vi "Find Test Cases.vi"(8 "error in (no error)":errorcluster, 10 "Project or Class Path":path, 11 "Test Finder In":refnum<class "Test Finder.lvclass">) -> (0 "error out":errorcluster, 3 "Test Finder Out":refnum<class "Test Finder.lvclass">)   [LabVIEW 2020, in "Test Finder.lvclass"]
uses:
  Test Finder.lvclass
  Test Finder.lvclass/Test Finder.ctl
  Test Case/LUnit Test Case.lvclass
  <vilib>/Utility/error.llb/Error Cluster From Error Code.vi
  <vilib>/ErrorRing/Error Ring.xnode
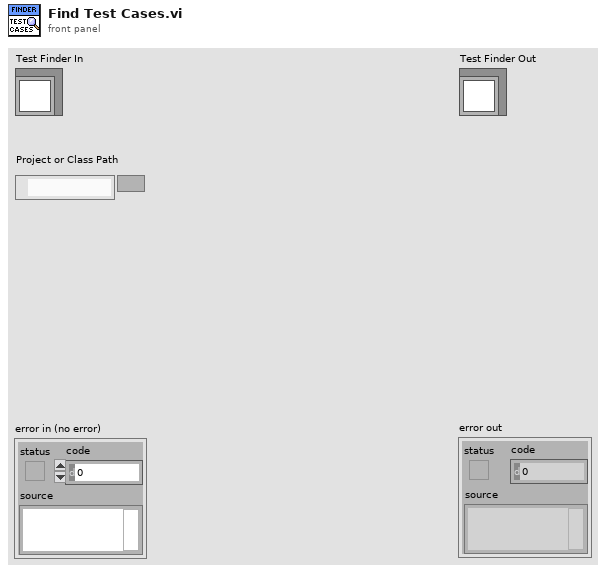
[diagram p1: front panel]
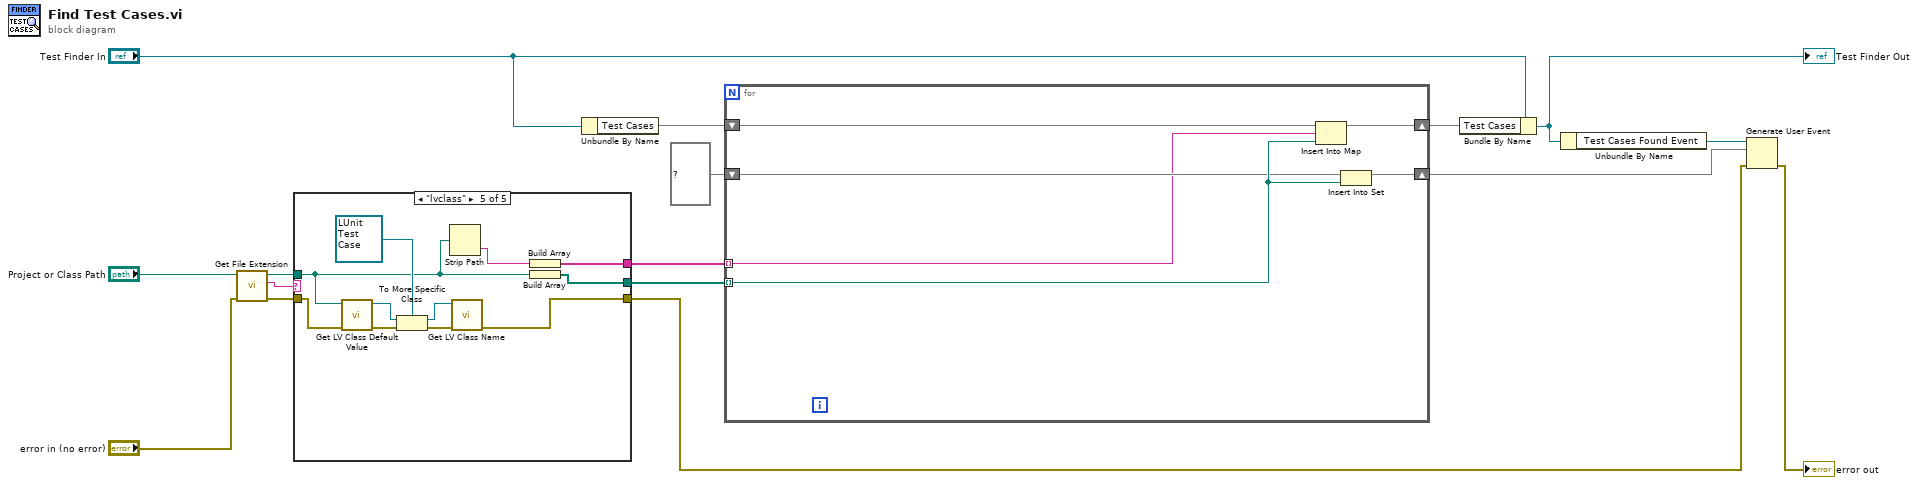
[diagram p0: block diagram]
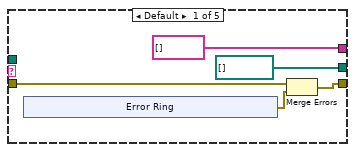
[diagram p2: hidden frame]
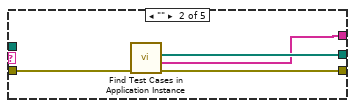
[diagram p3: hidden frame]
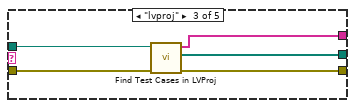
[diagram p4: hidden frame]
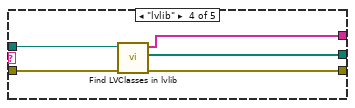
[diagram p5: hidden frame]
diagram:
  n1 = call <vilib>:"Get File Extension.vi"("error in (no error)"="error in (no error)", "file"="Project or Class Path") -> ("error out"=w13:errorcluster, "lowercase file extension"=w12:string, "dup file"=w15:path)  [unwired: 5 in, 2 out]
  n2 = case shown="\"lvclass\"" w12 {
    tunnel: w15 -> [_ _ w34 w39 w41]
    tunnel: w13 -> [w17 w27 w33 w38 w44]
    tunnel: [w18 w29 w31 w36 w43] -> w5
    tunnel: [path[] [] ("Class paths") w28 w32 w37 w50] -> w11
    tunnel: [string[] [] ("Classes in project") w26 w30 w35 w49] -> w1
    frame Default {
      n3 = xnode "Error Ring"() -> ("error out"=w21:errorcluster)
      n4 = Merge Errors(w17, w21) -> (w18:errorcluster)
    }
    frame "" {
      n5 = call "Find Test Cases in Application Instance.vi"("error in (no error)"=w27) -> ("error out"=w29:errorcluster, "Classes in App Instance"=w26:string[], "Class Paths"=w28:path[])  [unwired: 8 in]
    }
    frame "lvproj" {
      n6 = call "Find Test Cases in LVProj.vi"("error in (no error)"=w33, "Project Path"=w34) -> ("error out"=w31:errorcluster, "Class paths"=w32:path[], "Classes in project"=w30:string[])  [unwired: 7 in]
    }
    frame "lvlib" {
      n7 = call "Find LVClasses in lvlib.vi"("error in (no error)"=w38, "Library Path"=w39) -> ("error out"=w36:errorcluster, "Class paths"=w37:path[], "Classes in library"=w35:string[])  [unwired: 7 in]
    }
    frame "lvclass" {
      n8 = call <vilib>:"Get LV Class Default Value.vi"("error in (no error)"=w44, "class path"=w41) -> ("error out"=w48:errorcluster, "object"=w46:refnum<class>)  [unwired: 8 in]
      n9 = To More Specific Class(target class=refnum<class "LUnit Test Case.lvclass"> refnum ("LUnit Test Case.lvclass"), reference=w46, error in=w48) -> (specific class reference=w45:refnum<class "LUnit Test Case.lvclass">, error out=w47:errorcluster)
      n10 = Strip Path(path=w41) -> (name=w40:string)  [unwired: 1 out]
      n11 = call <vilib>:"Get LV Class Name.vi"("error in (no error)"=w47, "object"=w45) -> ("error out"=w43:errorcluster)  [unwired: 8 in, 1 out]
      n12 = Build Array(w40) -> (w49:string[])
      n13 = Build Array(w41) -> (w50:path[])
    }
  }
  n14 = Unbundle By Name("Test Finder In") -> ("Test Cases"=w9:map{string, path})
  n15 = for {
    tunnel: w11 -> [w54] mode=indexing
    shift-right: [w55] -> w8
    shift-left: w9 -> [w56]
    shift-right: [w53] -> w2
    shift-left: set{path} {} ("event data") -> [w52]
    tunnel: w1 -> [w51] mode=indexing
    n16 = Insert Into Map(map in=w56, key=w51, value=w54) -> (map out=w55:map{string, path})  [unwired: 2 out]
    n17 = Insert Into Set(10:w54, 11:w52) -> (3:w53:set{path})  [unwired: 1 out]
  }
  n18 = Bundle By Name(cluster="Test Finder In", "Test Cases"=w8) -> (w7:refnum<class "Test Finder.lvclass">)
  "Test Finder Out" <- w7
  n19 = Unbundle By Name(w7) -> ("Test Cases Found Event"=w6:refnum<user-event>)
  n20 = Generate User Event(user event=w6, event data cluster=w2, error in=w5) -> (error out=→"error out":errorcluster)  [unwired: 1 in, 1 out]
